vi "Set Window Time.vi"(7 "Ref Window Time":refnum<vi>, 8 "error in":errorcluster, 10 "Pulsar Handle":i16, 11 "OphirFastX (in)":refnum<k7>) -> (0 "error out":errorcluster, 3 "OphirFastX (out)":refnum<k7>)   [LabVIEW 2009]
panel:
  # "Guillaume Plateau - yguig2@yahoo.fr"
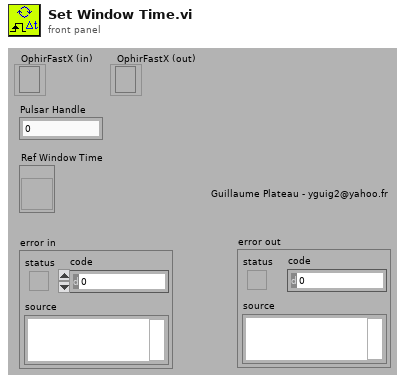
[diagram p1: front panel]
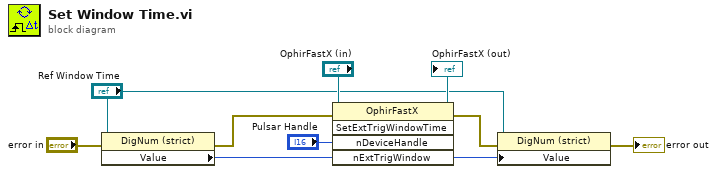
[diagram p0: block diagram]
diagram:
  n1 = property class="DigNum (strict)"(reference="Ref Window Time", error in="error in") -> (error out=w4:errorcluster, "Value"=w7:i32)  [unwired: 1 out]
  n2 = invoke class="OphirFastX" method="SetExtTrigWindowTime"(reference="OphirFastX (in)", error in=w4, "nDeviceHandle"="Pulsar Handle", "nExtTrigWindow"=w7) -> (reference out=→"OphirFastX (out)":refnum<k7>, error out=w3:errorcluster, "nExtTrigWindow"=w6:i16)  [unwired: 1 in, 2 out]
  n3 = property class="DigNum (strict)"(reference="Ref Window Time", error in=w3, "Value"=w6) -> (error out=→"error out":errorcluster)  [unwired: 1 out]
